vi "RRTAlgorithm.vi"(0 "Dest x,y":dbl[](array[numeric]), 1 "Robot":T1, 2 "WayPointProb":dbl, 3 "Path in \n(Smooth do Feedback Node)":dbl[][](array[numeric]), 4 "Step":dbl, 5 "GoalProb":dbl, 6 "Simple Path":dbl[][](array[numeric]), 7 "Ball":T6, 8 "Initial Pos x,y":dbl[](array[numeric]), 9 "our_robots":T1[](array[typedef]), 10 "Initial Pos 1,x,y,0":dbl[](array[numeric]), 11 "enemy_robots":T1[](array[typedef]), 13 "Field Geomtery":u32[](array[numeric])) -> (16 "Path":dbl[][](array[numeric]))   [LabVIEW 2017]
uses:
  kD-tree/KD-Tree.ctl
  kD-tree/Node.ctl
  Core/AI Ball.ctl
  Core/AI Robot.ctl
  Intel/Functions Enum.ctl
  Intel/AttackerStates.ctl
  PathDests.ctl
  PathDest.ctl
  <vilib>/Analysis/_algsub.llb/Real Vector Norm.vi
  <vilib>/Analysis/NI_AALPro.lvlib
panel:
  out "Elapsed Time (s)":dbl
  out "New KD-Tree":T7
  out "x > y? 2":bool
  out "Modulo":dbl
  in  "threshold":dbl=80.0
  out "Time has Elapsed":bool
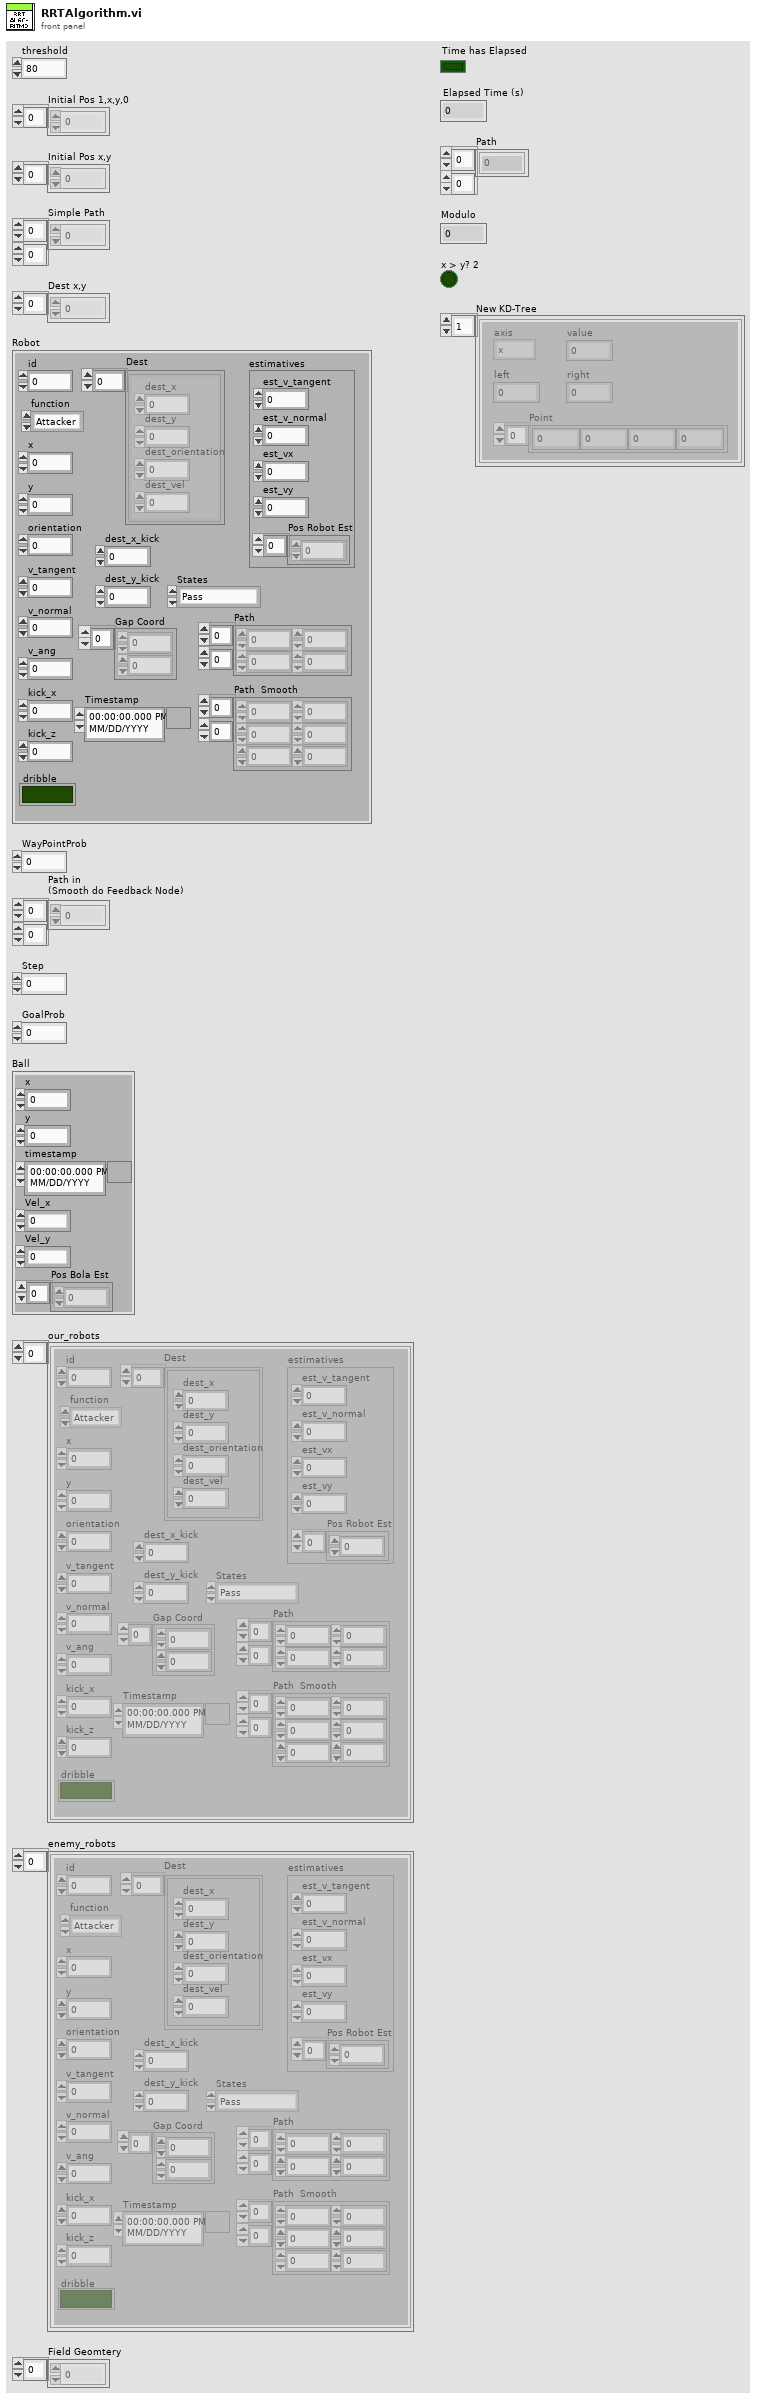
[diagram p1: front panel]
types:
  T1 = typedef "AI Robot.ctl" = cluster{"id":u32, "function":T2, "x":dbl, "y":dbl, "orientation":dbl, "v_tangent":dbl, "v_normal":dbl, "v_ang":dbl, "kick_x":dbl, "kick_z":dbl, "dribble":bool, "Timestamp":timestamp, "estimatives":cluster{"est_v_tangent":dbl, "est_v_normal":dbl, "est_vx":dbl, "est_vy":dbl, "Pos Robot Est":dbl[]}, "dest_x_kick":dbl, "dest_y_kick":dbl, "Gap Coord":dbl[], "States":T3, "Path ":dbl[][], "Path  Smooth":dbl[][], "Dest":T4}
  T2 = typedef "Functions Enum.ctl" = enum16{"Attacker", "Goalie", "Defender", "Striker", "Goto 0", "Dummy", "Kicker", "ZigZag 0", "ZigZag 1", "ZigZag 2", "ZigZag 3", "ZigZag 4", "ZigZag 5", "ZigZag 6", "ZigZag 7", "ZigZag 8", ""}
  T3 = typedef "AttackerStates.ctl" = enum16{"Pass", "GoToTangent", "BallGetting", "GoToKick", ""}
  T4 = typedef "PathDests.ctl" = T5[]
  T5 = typedef "PathDest.ctl" = cluster{"dest_x":dbl, "dest_y":dbl, "dest_orientation":dbl, "dest_vel":dbl}
  T6 = typedef "AI Ball.ctl" = cluster{"x":dbl, "y":dbl, "timestamp":timestamp, "Vel_x":dbl, "Vel_y":dbl, "Pos Bola Est":dbl[]}
  T7 = typedef "KD-Tree.ctl" = T8[]
  T8 = typedef "Node.ctl" = cluster{"axis":enum16{"null", "x", "y"}, "value":dbl, "left":dbl, "right":dbl, "Point":dbl[]}
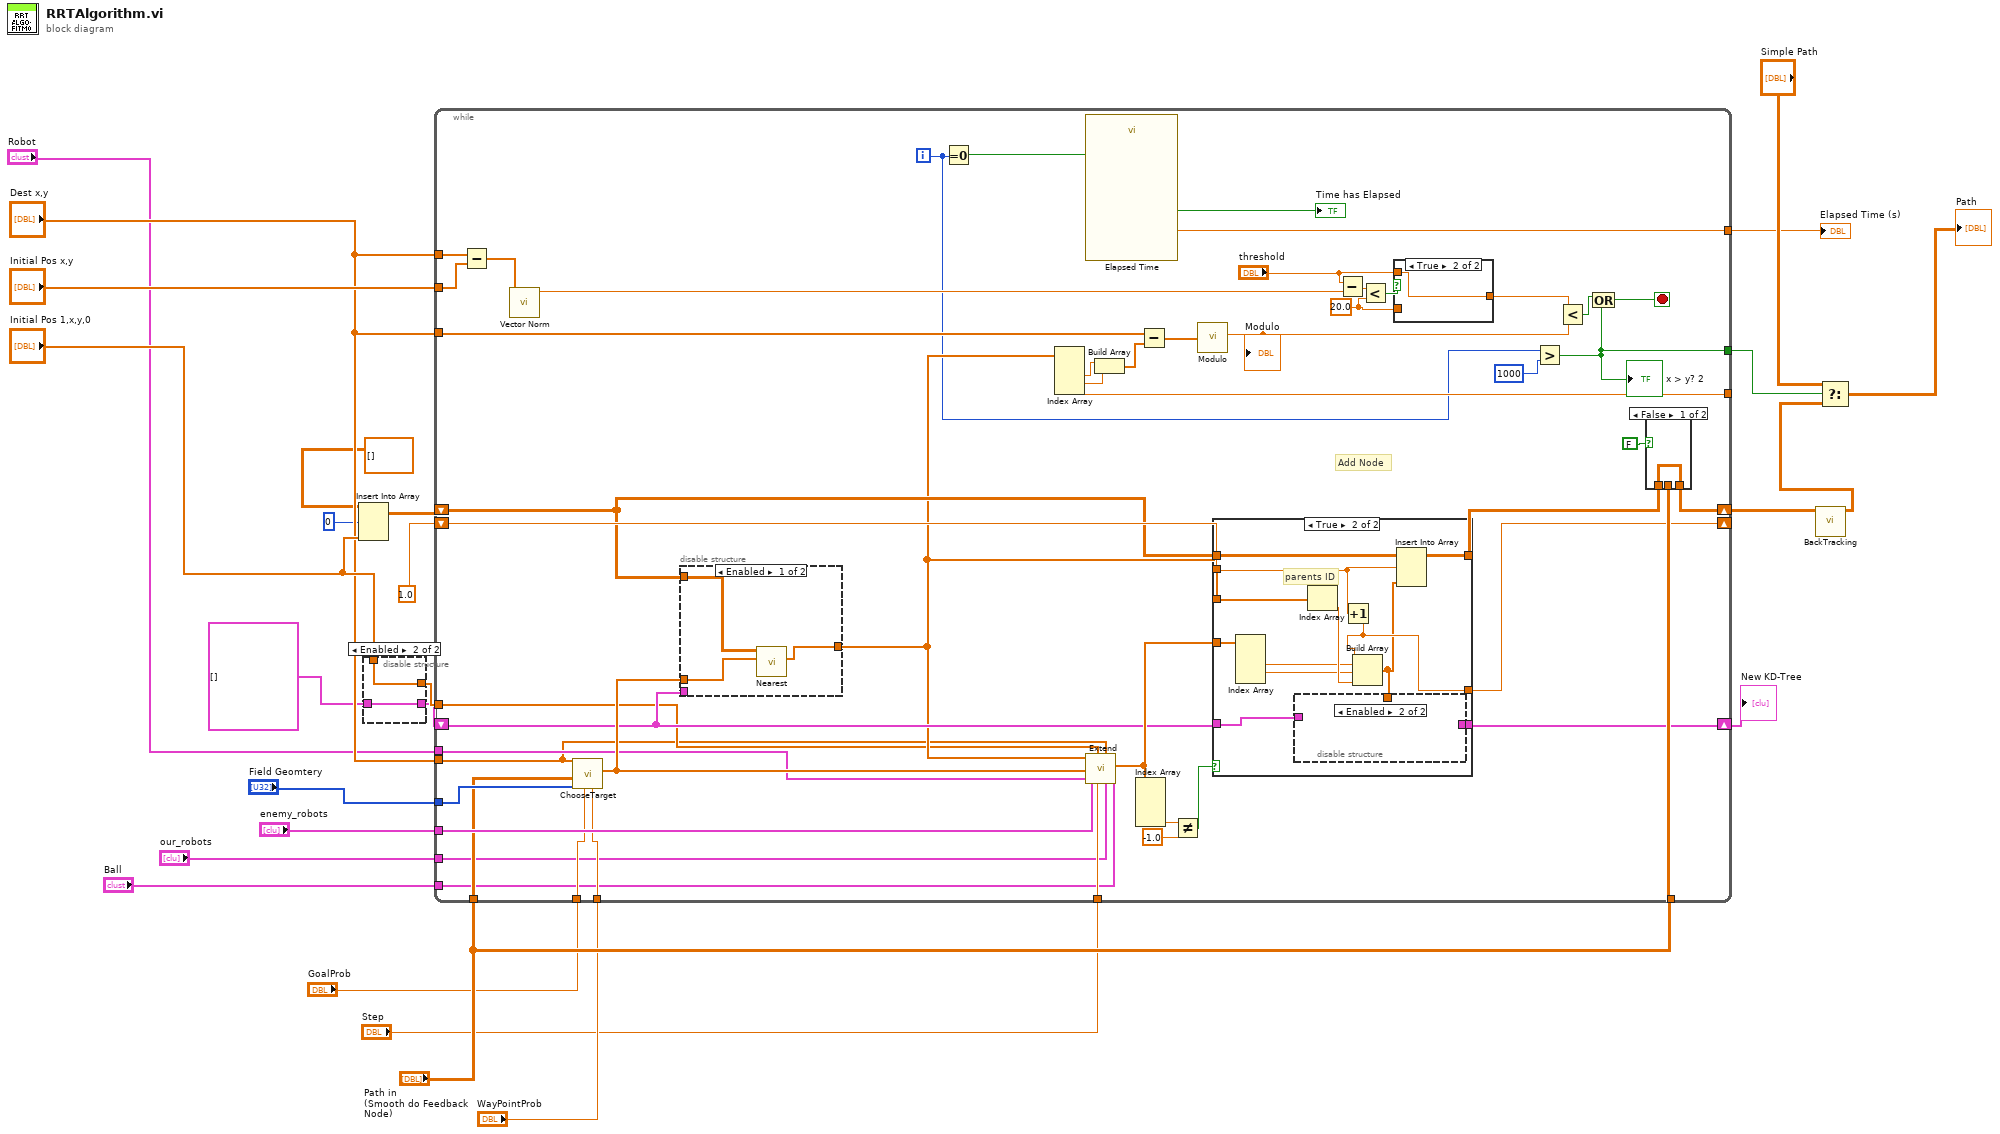
[diagram p0: block diagram]
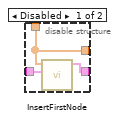
[diagram p2: hidden frame]
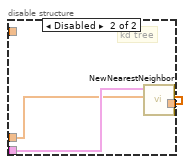
[diagram p3: hidden frame]
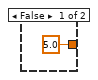
[diagram p4: hidden frame]
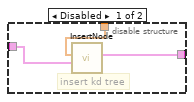
[diagram p7: hidden frame]
diagram:
  n1 = Insert Into Array(array=dbl[][] [] ("Pontos"), index (row)=0, new element="Initial Pos 1,x,y,0") -> (w3:dbl[][])  [unwired: 1 in]
  n2 = disable-structure shown="Enabled" {
    disable-tunnel: [w29 w31] -> w12
    disable-tunnel: T7 [] ("New KD-Tree") -> [w28 w31]
    disable-tunnel: "Initial Pos 1,x,y,0" -> [w27 w30]
    disable-tunnel: [w27 w30] -> w16
    frame Disabled {
      n3 = call "InsertFirstNode.vi"("New KD-Tree in"=w28, "Tree"=w27) -> ("New KD-Tree out"=w29:T7)  [unwired: 9 in]
    }
    frame Enabled {
    }
  }
  n4 = while {
    tunnel: "Dest x,y" -> [w80]
    tunnel: "Dest x,y" -> [w33]
    tunnel: "Field Geomtery" -> [w77]
    shift-right: [w61] -> w24
    shift-left: w3 -> [w60]
    tunnel: "enemy_robots" -> [w75]
    tunnel: "Step" -> [w74]
    shift-right: [w58] -> _
    shift-left: 1.0 -> [w65]
    tunnel: "Path in \n(Smooth do Feedback Node)" -> [w64]
    tunnel: "Path in \n(Smooth do Feedback Node)" -> [w63]
    tunnel: "GoalProb" -> [w56]
    tunnel: "WayPointProb" -> [w55]
    tunnel: [w53] -> _
    tunnel: "Dest x,y" -> [w52]
    shift-right: [w45] -> w11
    shift-left: w12 -> [w44]
    tunnel: [w42] -> w14
    tunnel: "Robot" -> [w40]
    tunnel: w16 -> [w39]
    tunnel: "Initial Pos x,y" -> [w38]
    tunnel: "our_robots" -> [w37]
    tunnel: "Ball" -> [w36]
    tunnel: [w32] -> w22
    i -> [w35]
    stop <- w69 stop-if-true
    w46 = 20.0 ("y")
    # "Add Node"
    n5 = Subtract(x=w52, y=w38) -> (x-y=w51:dbl[])
    n6 = call-poly <vilib>:"Vector Norm.vi"("Input Vector"=w51) -> ("norm"=w49:dbl)  [unwired: 9 in, 1 out]
    n7 = call "ChooseTarget.vi"("WayPointProb"=w55, "GoalProb"=w56, "Field Geometry"=w77, "WayPointCache"=w64, "Goal"=w33) -> ("Target"=w76:dbl[])  [unwired: 6 in]
    n8 = disable-structure shown="Enabled" {
      disable-tunnel: w76 -> [w84 w86]
      disable-tunnel: w60 -> [w83 _]
      disable-tunnel: w44 -> [_ w87]
      disable-tunnel: [w82 w85] -> w43
      frame Enabled {
        n9 = call "Nearest.vi"("Target"=w84, "Pontos"=w83) -> ("Nearest"=w82:dbl[])  [unwired: 9 in]
      }
      frame Disabled {
        # "kd tree"
        n10 = call "NewNearestNeighbor.vi"("q"=w86, "KD-Tree"=w87) -> ("Nearest"=w85:dbl[])  [unwired: 9 in]
      }
    }
    n11 = Equal To 0?(x=w35) -> (x = 0?=w41:bool)
    n12 = Index Array(array=w43) -> (element #2=w68:dbl, element #3=w67:dbl, element #4=w53:dbl)  [unwired: 4 in, 1 out]
    n13 = call "Elapsed Time"("Auto Reset"=w41) -> ("Elapsed Time (s)"=w42:dbl, "Time has Elapsed"=→"Time has Elapsed":bool)  [unwired: 11 in, 6 out]
    n14 = call "Extend.vi"("Ball"=w36, "our_robots"=w37, "Goal"=w33, "Step"=w74, "Initial State"=w39, "enemy_robots"=w75, "Robot in"=w40, "Target"=w76, "Nearest"=w43) -> ("New State"=w70:dbl[])  [unwired: 2 in]
    n15 = Build Array(w68, w67) -> (w66:dbl[])
    n16 = Index Array(array=w70) -> (element #4=w73:dbl)  [unwired: 4 in, 3 out]
    n17 = Subtract(x=w80, y=w66) -> (x-y=w81:dbl[])
    n18 = Not Equal?(x=w73, y=-1.0) -> (x != y?=w71:bool)
    n19 = call "Modulo.vi"("2D vector"=w81) -> ("Modulo"=w79:dbl)  [unwired: 10 in]
    "Modulo" <- w79
    n20 = case shown="True" w71 {
      tunnel: w60 -> [w94 w106]
      tunnel: [w94 w102] -> w62
      tunnel: w70 -> [_ w105]
      tunnel: w65 -> [w93 w101]
      tunnel: w43 -> [_ w104]
      tunnel: [w93 w96] -> w58
      tunnel: [w92 w100] -> w45
      tunnel: w44 -> [w92 w99]
      frame False {
      }
      frame True {
        # "parents ID"
        n21 = Index Array(array=w105) -> (element #2=w98:dbl, element #3=w97:dbl)  [unwired: 4 in, 2 out]
        n22 = Index Array(array=w104) -> (element=w103:dbl)  [unwired: 1 in]
        n23 = Increment(x=w101) -> (x+1=w96:dbl)
        n24 = Build Array(w96, w98, w97, w103) -> (w95:dbl[])
        n25 = disable-structure shown="Enabled" {
          disable-tunnel: [w109 _] -> w100
          disable-tunnel: w99 -> [w108 _]
          disable-tunnel: w95 -> [w107 _]
          frame Disabled {
            # "insert kd tree"
            n26 = call "InsertNode.vi"("KD-Tree"=w108, "New Node"=w107) -> ("New KD-Tree"=w109:T7)  [unwired: 9 in]
          }
          frame Enabled {
          }
        }
        n27 = Insert Into Array(array=w106, index (row)=w101, new element=w95) -> (w102:dbl[][])  [unwired: 1 in]
      }
    }
    n28 = Subtract(x="threshold", y=w49) -> (x-y=w47:dbl)
    n29 = Less?(x=w47, y=w46) -> (x < y?=w48:bool)
    n30 = case shown="True" w48 {
      tunnel: [5.0 ("threshold") w89] -> w78
      tunnel: "threshold" -> [_ w89]
      tunnel: w46 -> [_ _]
      frame False {
      }
      frame True {
      }
    }
    n31 = Greater?(x=w35, y=1000) -> (0:w32:bool)
    "x > y? 2" <- w32
    n32 = Less?(x=w79, y=w78) -> (x < y?=w54:bool)
    n33 = Compound Arithmetic op=OR(w54, w32) -> (w69:bool)
    n34 = case shown="False" FALSE {
      tunnel: w63 -> [_ w91]
      tunnel: [w90 w91] -> w61
      tunnel: w62 -> [w90 _]
      frame False {
      }
      frame True {
      }
    }
  }
  "New KD-Tree" <- w11
  "Elapsed Time (s)" <- w14
  n35 = call "BackTracking.vi"("Pontos"=w24) -> ("Path"=w26:dbl[][])  [unwired: 9 in, 1 out]
  n36 = Select(t="Simple Path", s=w22, f=w26) -> (s? t:f=→"Path":dbl[][])
